vi "Create Pattern Script(DataCapure).vi"(7 "Num of Cycles":i8, 8 "error in (no error)":errorcluster, 10 "Opcode":string, 11 "BurstLength":T1) -> (0 "error out":errorcluster, 3 "String":string)   [LabVIEW 2018, in "BML_Frame_Root.lvclass"]
uses:
  BML_Frame_Root.lvclass
  Config_Read/BurstLength.ctl
  Config_Read/Config_Read_BML.lvclass
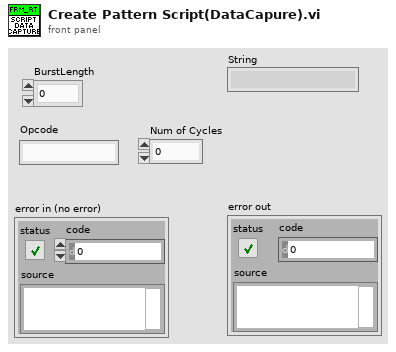
[diagram p1: front panel]
types:
  T1 = typedef "Config_Read_BML.lvclass/BurstLength.ctl" = enum8{"0", "2", "3", "4", "5", "8", "16", "32"}
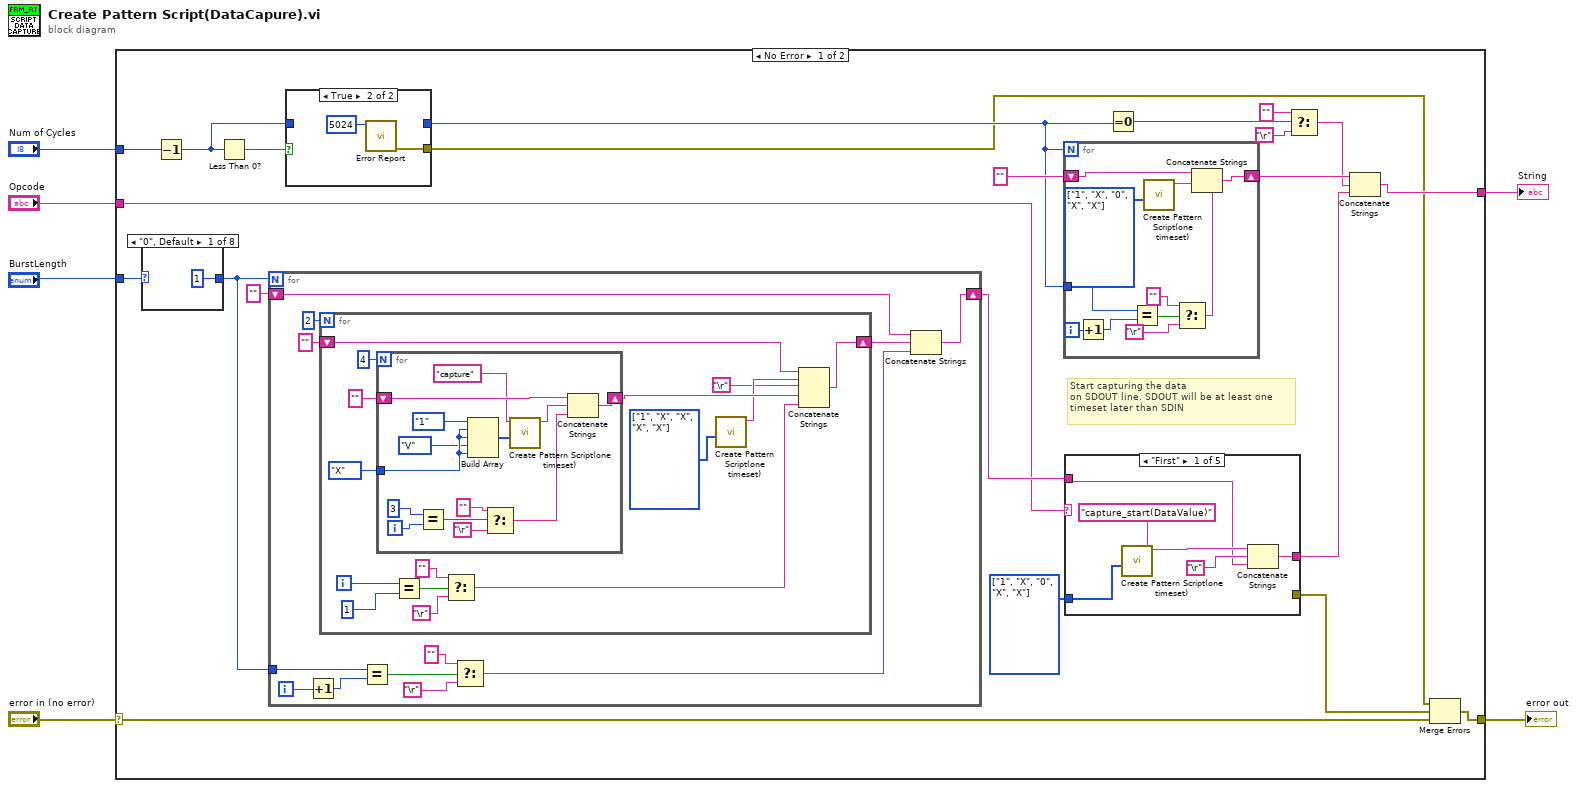
[diagram p0: block diagram]
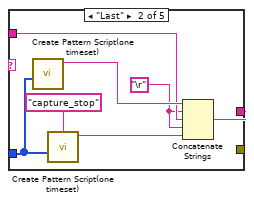
[diagram p3: hidden frame]
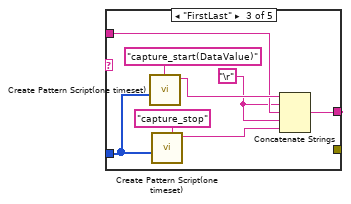
[diagram p4: hidden frame]
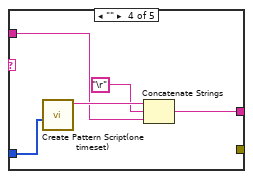
[diagram p5: hidden frame]
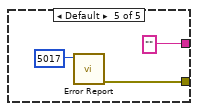
[diagram p6: hidden frame]
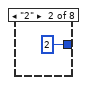
[diagram p7: hidden frame]
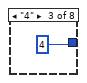
[diagram p8: hidden frame]
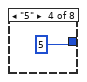
[diagram p9: hidden frame]
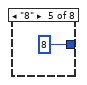
[diagram p10: hidden frame]
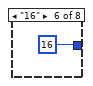
[diagram p11: hidden frame]
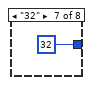
[diagram p12: hidden frame]
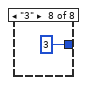
[diagram p13: hidden frame]
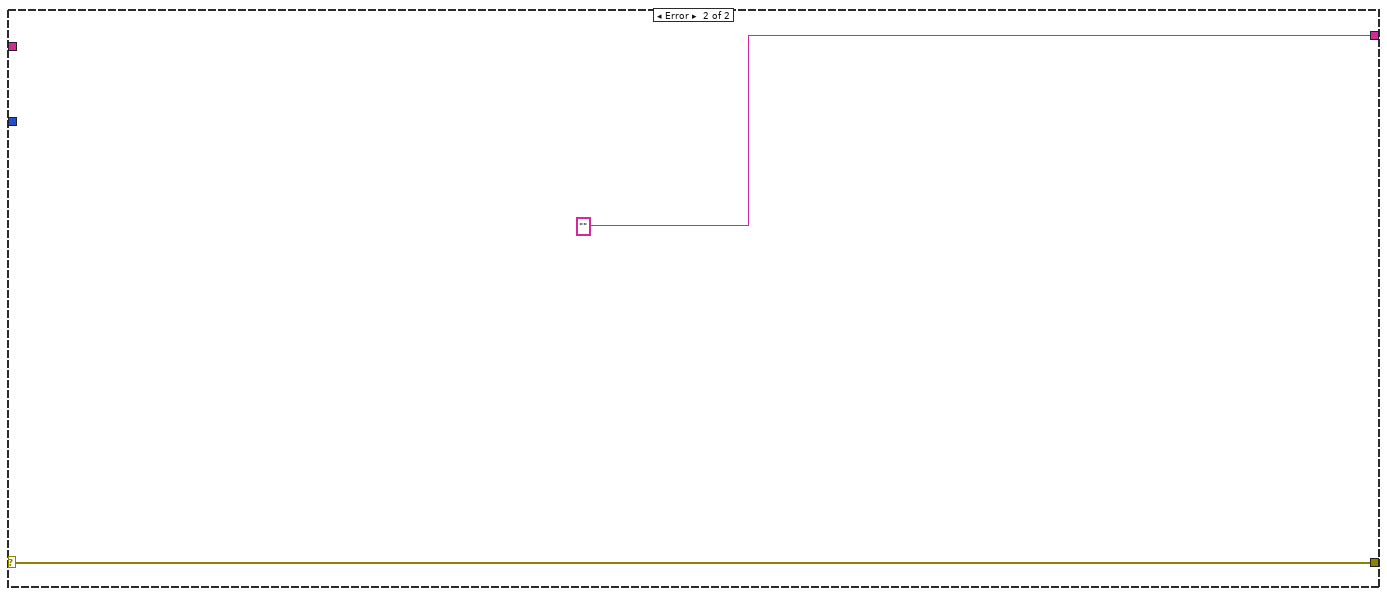
[diagram p14: hidden frame]
diagram:
  n1 = case shown="No Error" "error in (no error)" {
    selector: "error in (no error)" -> [w22 w121]
    tunnel: [w8 ""] -> w5
    tunnel: [w21 w121] -> w4
    tunnel: "BurstLength" -> [w27 _]
    tunnel: "Opcode" -> [w23 _]
    tunnel: "Num of Cycles" -> [w19 _]
    frame No Error {
      w25 = enum16{"0", "1", "L", "H", "X", "V", "D", "M"}[] [enum."1", enum."X", enum."0", enum."X", enum."X"] items=["0", "1", "L", "H", "X", "V", "D", "M"] ("PinState")
      # "Start capturing the data\non SDOUT line. SDOUT will be at least one \ntimeset later than SDIN"
      n2 = case shown="\"0\", Default" w27 {
        tunnel: [1 ("y") 2 ("y") 4 ("y") 5 ("y") 8 ("y") 16 ("y") 32 ("y") 3 ("y")] -> w26
        frame "0", Default {
        }
        frame "2" {
        }
        frame "4" {
        }
        frame "5" {
        }
        frame "8" {
        }
        frame "16" {
        }
        frame "32" {
        }
        frame "3" {
        }
      }
      n3 = Decrement(x=w19) -> (x-1=w16:i8)
      n4 = Less Than 0?(x=w16) -> (x < 0?=w17:bool)
      n5 = for {
        N: w26 -> [_]
        shift-right: [w82] -> w24
        shift-left: "" -> [w81]
        tunnel: w26 -> [w80]
        i -> [w89]
        n6 = Increment(x=w89) -> (x+1=w88:i32)
        n7 = for {
          N: 2 -> [_]
          shift-right: [w98] -> w84
          shift-left: "" -> [w95]
          i -> [w105]
          w94 = enum16{"0", "1", "L", "H", "X", "V", "D", "M"}[] [enum."1", enum."X", enum."X", enum."X", enum."X"] items=["0", "1", "L", "H", "X", "V", "D", "M"] ("PinState")
          n8 = for {
            N: 4 -> [_]
            shift-right: [w115] -> w100
            shift-left: "" -> [w108]
            tunnel: enum16{"0", "1", "L", "H", "X", "V", "D", "M"}."X" ("element") -> [w110]
            i -> [w120]
            n9 = Equal?(x=3, y=w120) -> (x = y?=w118:bool)
            n10 = Build Array(enum16{"0", "1", "L", "H", "X", "V", "D", "M"}."1" ("element"), w110, w110, enum16{"0", "1", "L", "H", "X", "V", "D", "M"}."V" ("PinState"), w110) -> (w113:enum16{"0", "1", "L", "H", "X", "V", "D", "M"}[])
            n11 = Select(t="", s=w118, f="\r") -> (s? t:f=w114:string)
            n12 = call "Create Pattern Script(one timeset).vi"("PinState"=w113, "opcode"="capture") -> ("string out"=w112:string)  [unwired: 9 in]
            n13 = Concatenate Strings(w108, w112, w114) -> (w115:string)
          }
          n14 = Equal?(x=w105, y=1) -> (x = y?=w103:bool)
          n15 = Select(t="", s=w103, f="\r") -> (s? t:f=w99:string)
          n16 = call "Create Pattern Script(one timeset).vi"("PinState"=w94) -> ("string out"=w93:string)  [unwired: 10 in]
          n17 = Concatenate Strings(w95, w93, "\r", w100, w99) -> (w98:string)
        }
        n18 = Equal?(x=w80, y=w88) -> (x = y?=w85:bool)
        n19 = Select(t="", s=w85, f="\r") -> (s? t:f=w83:string)
        n20 = Concatenate Strings(w81, w84, w83) -> (w82:string)
      }
      n21 = case shown="True" w17 {
        tunnel: w16 -> [w29 _]
        tunnel: [w29 _] -> w14
        tunnel: [_ w30] -> w7
        frame False {
        }
        frame True {
          n22 = call "Error Report.vi"("Error Code"=i16 5024) -> ("error out"=w30:errorcluster)  [unwired: 10 in]
        }
      }
      n23 = for {
        N: w14 -> [_]
        shift-right: [w40] -> w15
        shift-left: "" -> [w39]
        tunnel: w14 -> [w33]
        i -> [w34]
        w42 = enum16{"0", "1", "L", "H", "X", "V", "D", "M"}[] [enum."1", enum."X", enum."0", enum."X", enum."X"] items=["0", "1", "L", "H", "X", "V", "D", "M"] ("PinState")
        n24 = Increment(x=w34) -> (x+1=w38:i32)
        n25 = Equal?(x=w33, y=w38) -> (x = y?=w35:bool)
        n26 = call "Create Pattern Script(one timeset).vi"("PinState"=w42) -> ("string out"=w41:string)  [unwired: 10 in]
        n27 = Select(t="", s=w35, f="\r") -> (s? t:f=w32:string)
        n28 = Concatenate Strings(w39, w41, w32) -> (w40:string)
      }
      n29 = case shown="\"First\"" w23 {
        tunnel: w25 -> [w48 w50 w58 w64 _]
        tunnel: w24 -> [w44 w54 w62 w67 _]
        tunnel: [w43 w53 w61 w66 ""] -> w9
        tunnel: [_ _ _ _ w69] -> w20
        frame "First" {
          n30 = call "Create Pattern Script(one timeset).vi"("PinState"=w48, "opcode"="capture_start(DataValue)") -> ("string out"=w46:string)  [unwired: 9 in]
          n31 = Concatenate Strings(w46, "\r", w44) -> (w43:string)
        }
        frame "Last" {
          w52 = "\r"
          n32 = call "Create Pattern Script(one timeset).vi"("PinState"=w50) -> ("string out"=w55:string)  [unwired: 10 in]
          n33 = call "Create Pattern Script(one timeset).vi"("PinState"=w50, "opcode"="capture_stop") -> ("string out"=w49:string)  [unwired: 9 in]
          n34 = Concatenate Strings(w55, w52, w54, w52, w49) -> (w53:string)
        }
        frame "FirstLast" {
          w60 = "\r"
          n35 = call "Create Pattern Script(one timeset).vi"("PinState"=w58, "opcode"="capture_start(DataValue)") -> ("string out"=w63:string)  [unwired: 9 in]
          n36 = call "Create Pattern Script(one timeset).vi"("PinState"=w58, "opcode"="capture_stop") -> ("string out"=w57:string)  [unwired: 9 in]
          n37 = Concatenate Strings(w63, w60, w62, w60, w57) -> (w61:string)
        }
        frame "" {
          n38 = call "Create Pattern Script(one timeset).vi"("PinState"=w64) -> ("string out"=w68:string)  [unwired: 10 in]
          n39 = Concatenate Strings(w68, "\r", w67) -> (w66:string)
        }
        frame Default {
          n40 = call "Error Report.vi"("Error Code"=i16 5017) -> ("error out"=w69:errorcluster)  [unwired: 10 in]
        }
      }
      n41 = Equal To 0?(x=w14) -> (x = 0?=w13:bool)
      n42 = Select(t="", s=w13, f="\r") -> (s? t:f=w10:string)
      n43 = Concatenate Strings(w15, w10, w9) -> (w8:string)
      n44 = Merge Errors(w7, w20, w22) -> (w21:errorcluster)
    }
    frame Error {
    }
  }
  "String" <- w5
  "error out" <- w4
